vi "Open My Data CSV.vi"(5 "Comment":string, 7 "Time Stamp":timestamp, 8 "error in":errorcluster, 11 "file path":path) -> (0 "error out":errorcluster, 3 "refnum out":refnum<file>)   [LabVIEW 2014]
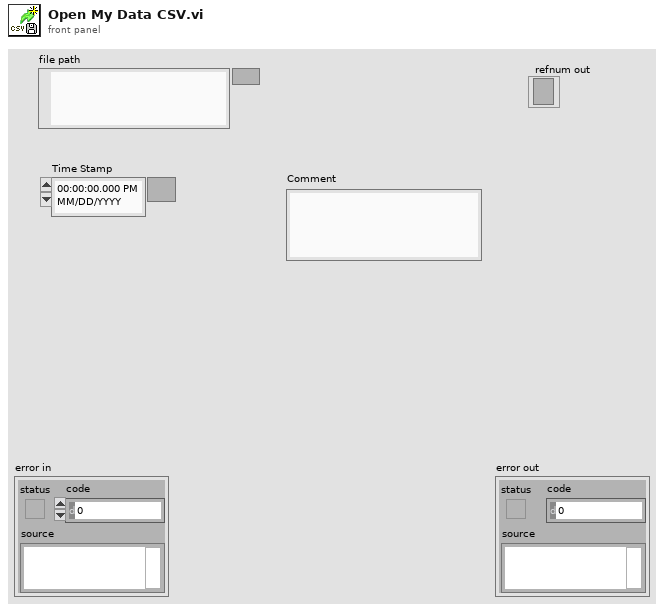
[diagram p1: front panel]
types:
  T1 = enum16{"open", "replace", "create", "open or create", "replace or create", "replace or create with confirmation"}
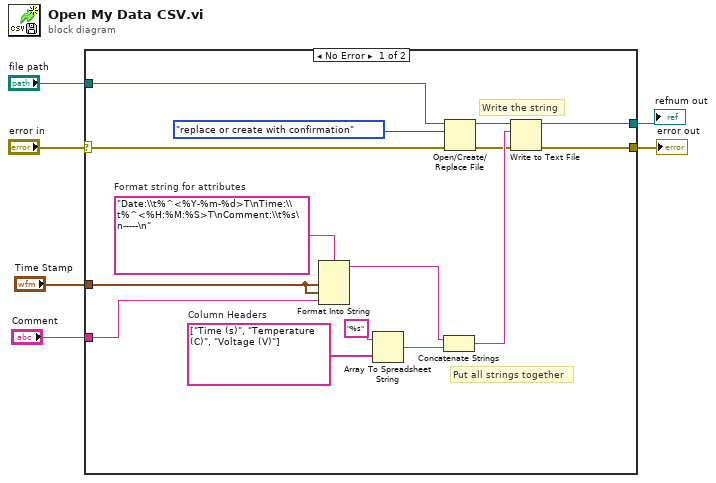
[diagram p0: block diagram]
diagram:
  n1 = case shown="No Error" "error in" {
    selector: "error in" -> [w9 w22]
    tunnel: [w17 w22] -> w6
    tunnel: "file path" -> [w11 _]
    tunnel: "Time Stamp" -> [w15 _]
    tunnel: "Comment" -> [w14 _]
    tunnel: [w12 _] -> w1
    frame No Error {
      w16 = "Date:\\t%^<%Y-%m-%d>T\nTime:\\t%^<%H:%M:%S>T\nComment:\\t%s\n-----\n"  # Format string for attributes
      w21 = string[] ["Time (s)", "Temperature (C)", "Voltage (V)"]  # Column Headers
      # "Write the string"
      # "Put all strings together"
      n2 = Format Into String(format string=w16, w15, w15, w14) -> (resulting string=w13:string)  [unwired: 2 in, 1 out]
      n3 = Array To Spreadsheet String(array=w21, 3:"%s" ("format string")) -> (spreadsheet string=w20:string)  [unwired: 1 in]
      n4 = Concatenate Strings(w13, w20) -> (w19:string)
      n5 = Open/Create/Replace File(file path (use dialog)=w11, error in=w9, operation (0:open)=T1."replace or create with confirmation") -> (refnum out=w10:refnum<file>, error out=w8:errorcluster)  [unwired: 3 in, 1 out]
      n6 = Write to Text File(file (use dialog)=w10, text=w19, error in=w8) -> (refnum out=w12:refnum<file>, error out=w17:errorcluster)  [unwired: 1 in, 1 out]
    }
    frame Error {
      # "Wire previous error through"
    }
  }
  "error out" <- w6
  "refnum out" <- w1
